vi "Read Multi Value as Binary.vi"(6 "byte order":T1(ring), 8 "error in (no error)":errorcluster, 10 "Tag":string[](array[string]), 11 "Var Bus in":refnum<class "Omni_Bus.lvclass">) -> (0 "error out":errorcluster, 2 "Binary":string[](array[string]), 3 "Var Bus out":refnum<class "Omni_Bus.lvclass">)   [LabVIEW 2021, in "Omni_Bus.lvclass"]
uses:
  Omni_Bus.lvclass
  Omni_Bus.lvclass/Omni_Bus.ctl
  <vilib>/TSA/Abstract Data Classes/Abs_Types/Value/Abs_Value.lvclass
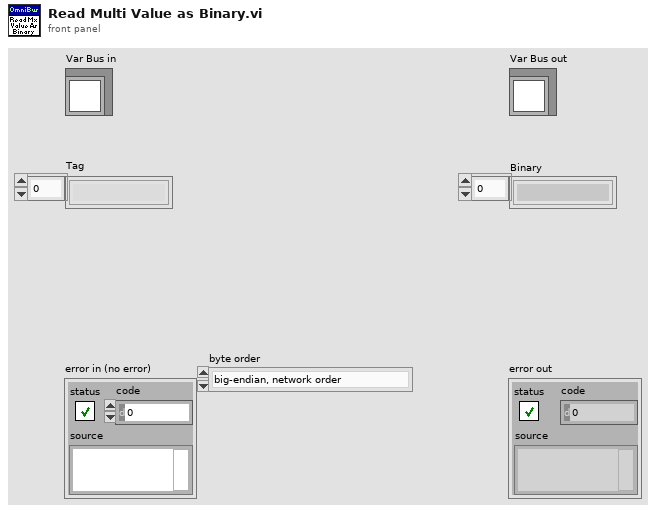
[diagram p1: front panel]
types:
  T1 = enum16{"big-endian, network order", "native, host order", "little-endian"}
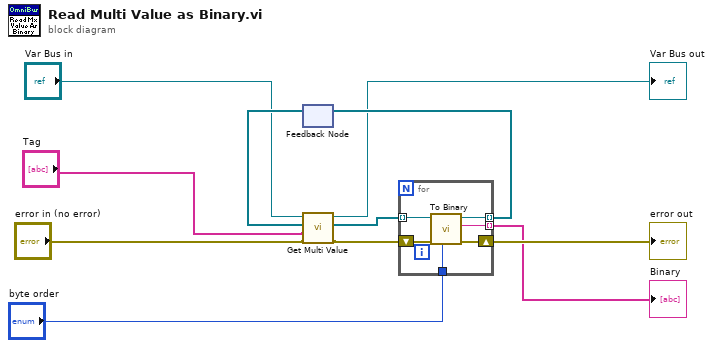
[diagram p0: block diagram]
diagram:
  n1 = feedback #1() -> (w4:refnum<class "Abs_Value.lvclass">[])  [unwired: 1 in]
  n2 = call-dynamic "Get Multi Value.vi"("error in (no error)"="error in (no error)", "Tag"="Tag", "Value Type"=w4, "Var Bus in"="Var Bus in") -> ("error out"=w8:errorcluster, "Value Out"=w7:refnum<class "Abs_Value.lvclass">[], "Var Bus out"=→"Var Bus out":refnum<class "Omni_Bus.lvclass">)  [unwired: 5 in]
  n3 = for {
    tunnel: [w16] -> w10 mode=indexing
    tunnel: [w15] -> w9 mode=indexing
    tunnel: w7 -> [w13] mode=indexing
    tunnel: "byte order" -> [w12]
    shift-right: [w17] -> w11
    shift-left: w8 -> [w14]
    n4 = call-dynamic "To Binary.vi"("byte order"=w12, "error in (no error)"=w14, "Type in"=w13) -> ("error out"=w17:errorcluster, "Binary"=w16:string, "Type out"=w15:refnum<class "Abs_Value.lvclass">)  [unwired: 6 in]
  }
  "error out" <- w11
  "Binary" <- w10
  n5 = feedback-in #1(w9) -> ()
